vi "3458A Initiate Digitizing Process.vi"(8 "error in":errorcluster, 11 "session in":T1 {"channels"."Range [Vpk]" min=0.0}) -> (0 "error out":errorcluster, 3 "session out":T1 {"channels"."Range [Vpk]" min=0.0})   [LabVIEW 2018, in "3458A Virtual Digitizer.lvlib"]
doc: "Initiates acquisition for both single shot and streaming modes. It creates data queues and starts digitizing processes, one for each channel. If succeds the process immediatelly starts digitizing (after trigger event occures) and starts filling the queues with data. So this VI must be immediatelly followed by fetch loop that takes out data from the queue! This may be called repeatedely without calling 'Setup' function if multiple records are required with identical configuration."
uses:
  3458A Virtual Digitizer.lvlib
  3458A Digitizer Session.ctl
  3458A Virtual Channel Config.ctl
  Counter/Counter Session.ctl
  Counter/Counter Type.ctl
  AWG/AWG Session.ctl
  AWG/AWG Type.ctl
  3458A Sync Mode.ctl
  3458A Idn Mode.ctl
  3458A Digitizing Low Levels/Configure/Sampling Mode.ctl
  3458A Digitizing Process Options.ctl
  3458A Data Packet.ctl
  3458A Aux Record Data.ctl
  3458A Digitizing Low Levels/Configure/Level Setup.ctl
  3458A Digitizing Low Levels/Configure/First Sample Trigger.ctl
  3458A Aperture Selection Mode.ctl
  AWG/AWG.lvlib
  Counter/Counter.lvlib
  3458A Digitizing Low Levels/3458A Digitizing Low Levels.lvlib
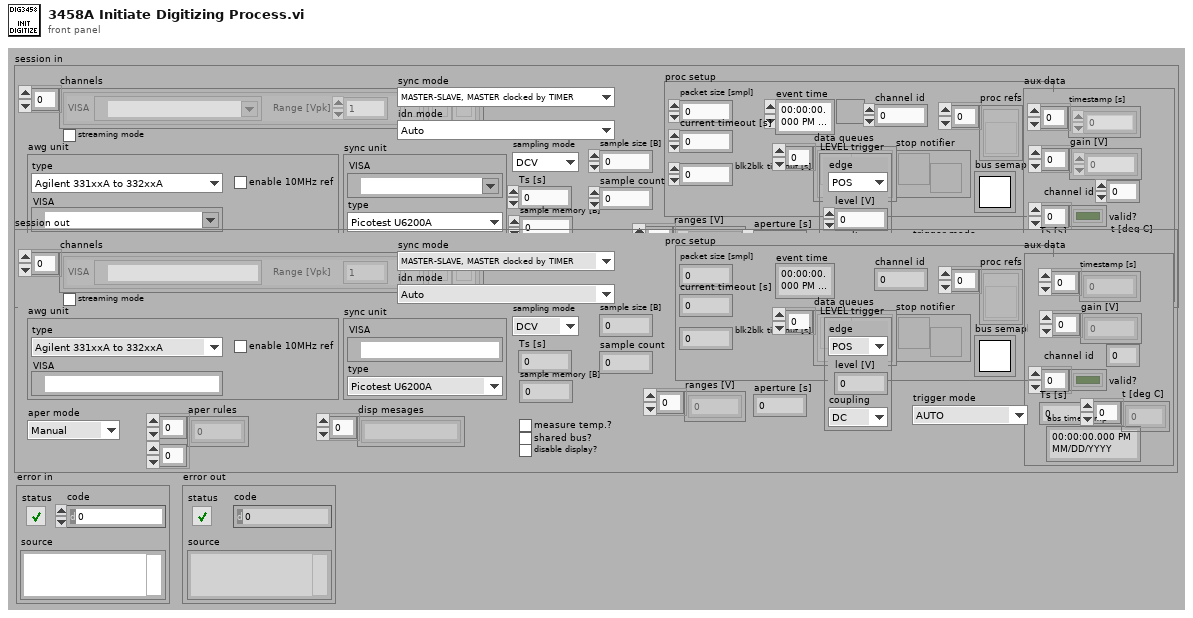
[diagram p1: front panel]
types:
  T1 = typedef "3458A Virtual Digitizer.lvlib/3458A Digitizer Session.ctl" = cluster{"channels":T2[], "sync unit":T3, "awg unit":T5, "sync mode":T7, "streaming mode":bool, "idn mode":T8, "sampling mode":T9, "Ts [s]":dbl, "sample memory [B]":i32, "proc setup":T10, "sample size [B]":i32, "sample count":i32, "aux data":T12, "ranges [V]":dbl[], "aperture [s]":dbl, "LEVEL trigger":T13, "trigger mode":T14, "measure temp.?":bool, "disp mesages":string[], "shared bus?":bool, "disable display?":bool, "aper mode":T15, "aper rules":dbl[][]}
  T2 = typedef "3458A Virtual Digitizer.lvlib/3458A Virtual Channel Config.ctl" = cluster{"VISA":refnum<visa-resource-name>, "Range [Vpk]":dbl, "btn clr":bool, "btn up":bool, "btn down":bool}
  T3 = typedef "Counter.lvlib/Counter Session.ctl" = cluster{"VISA":refnum<visa-resource-name>, "type":T4}
  T4 = typedef "Counter.lvlib/Counter Type.ctl" = enum16{"Picotest U6200A", "dummy"}
  T5 = typedef "AWG.lvlib/AWG Session.ctl" = cluster{"type":T6, "VISA":refnum<visa-resource-name>, "enable 10MHz ref":bool}
  T6 = typedef "AWG.lvlib/AWG Type.ctl" = enum16{"Agilent 331xxA to 332xxA", "Agilent 335xxA to 336xxA", "Tektronix AFG3101C", "dummy"}
  T7 = typedef "3458A Virtual Digitizer.lvlib/3458A Sync Mode.ctl" = enum16{"MASTER-SLAVE, MASTER clocked by TIMER", "MASTER-SLAVE, MASTER clocked by AWG", "ALL clocked by AWG", "MASTER-SLAVE, ALL clocked by TIMER", "ALL clocked by AWG with DFLL"}
  T8 = typedef "3458A Virtual Digitizer.lvlib/3458A Idn Mode.ctl" = enum16{"Auto", "Sequential (chn A, chn B, ...)", "From calibration string"}
  T9 = typedef "3458A Virtual Digitizer.lvlib/3458A Digitizing Low Levels.lvlib/Sampling Mode.ctl" = enum16{"DCV", "DSDC", "DSAC"}
  T10 = typedef "3458A Virtual Digitizer.lvlib/3458A Digitizing Process Options.ctl" = cluster{"channel id":i32, "packet size [smpl]":i32, "current timeout [s]":dbl, "blk2blk timeout [s]":dbl, "event time":timestamp, "stop notifier":refnum<notifier>, "data queues":refnum<queue>[], "proc refs":refnum<vi>[], "bus semaphore":T11}
  T11 = typedef "Semaphore RefNum" = refnum<k1>
  T12 = typedef "3458A Virtual Digitizer.lvlib/3458A Aux Record Data.ctl" = cluster{"channel id":i32, "valid?":bool[], "gain [V]":dbl[], "timestamp [s]":dbl[], "Ts [s]":dbl, "abs timestamp":timestamp, "t [deg C]":dbl[]}
  T13 = typedef "3458A Virtual Digitizer.lvlib/3458A Digitizing Low Levels.lvlib/Level Setup.ctl" = cluster{"edge":enum16{"POS", "NEG"}, "level [V]":dbl, "coupling":enum16{"DC", "AC"}}
  T14 = typedef "3458A Virtual Digitizer.lvlib/3458A Digitizing Low Levels.lvlib/First Sample Trigger.ctl" = enum16{"AUTO", "EXT", "SYN", "SGL", "HOLD", "LEVEL"}
  T15 = typedef "3458A Virtual Digitizer.lvlib/3458A Aperture Selection Mode.ctl" = enum16{"Manual", "Maximum", "Table"}
  T16 = typedef "3458A Virtual Digitizer.lvlib/3458A Data Packet.ctl" = cluster{"data":i32[][], "offset [smpl]":i32, "count [smpl]":i32, "all done?":bool, "sampling?":bool, "queue buffer [%]":dbl, "valid?":bool}
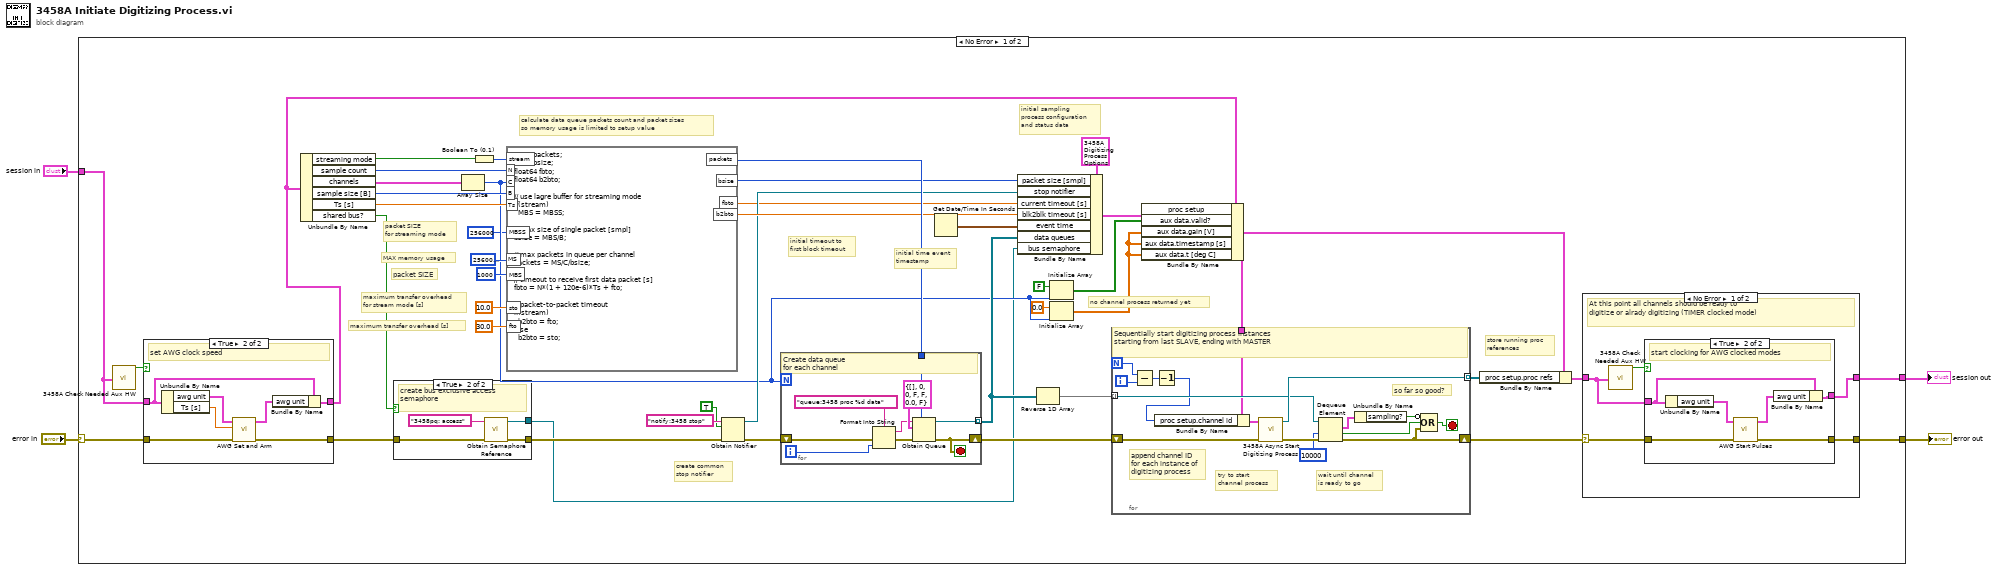
[diagram p0: block diagram]
diagram:
  n1 = case shown="No Error" "error in" {
    selector: "error in" -> [w8 w104]
    tunnel: [w24 w104] -> w4
    tunnel: "session in" -> [w7 w103]
    tunnel: [w23 w103] -> w2
    frame No Error {
      # "packet SIZE\nfor streaming mode"
      # "no channel process returned yet"
      # "initial time event\ntimestamp"
      # "maximum transfer overhead\nfor stream mode [s]"
      # "store running proc\nreferences"
      # "create common\nstop notifier"
      # "initial timeout to\nfirst block timeout"
      # "maximum transfer overhead [s]"
      # "initial sampling\nprocess configuration\nand status data"
      # "calculate data queue packets count and packet sizes\nso memory usage is limited to setup value"
      # "packet SIZE"
      # "MAX memory usage"
      n2 = call "3458A Check Needed Aux HW.vi"("digitizer session"=w7) -> ("uses AWG clocking?"=w6:bool)  [unwired: 13 in, 5 out]
      n3 = case shown="True" w6 {
        tunnel: w8 -> [w49 w57]
        tunnel: w7 -> [w50 w54]
        tunnel: [w49 w53] -> w9
        tunnel: [w50 w52] -> w5
        frame False {
          # "do nothing for TIMER clocked modes"
        }
        frame True {
          # "set AWG clock speed"
          n4 = Unbundle By Name(w54) -> ("awg unit"=w56:T5, "Ts [s]"=w51:dbl)
          n5 = call "AWG Set and Arm.vi"("error in (no error)"=w57, "T [s] (1ms)"=w51, "awg session in"=w56) -> ("error out"=w53:errorcluster, "awg session out"=w55:T5)  [unwired: 7 in]
          n6 = Bundle By Name(cluster=w54, "awg unit"=w55) -> (w52:T1)
        }
      }
      n7 = Unbundle By Name(w5) -> ("streaming mode"=w47:bool, "sample count"=w45:i32, "channels"=w44:T2[], "sample size [B]"=w22:i32, "Ts [s]"=w21:dbl, "shared bus?"=w12:bool)
      n8 = case shown="True" w12 {
        tunnel: w9 -> [w58 w62]
        tunnel: [w58 w61] -> w13
        tunnel: [_ w59] -> w11
        frame False {
        }
        frame True {
          # "create bus exclusive access\nsemaphore"
          n9 = call <vilib>:"Obtain Semaphore Reference.vi"("error in (no error)"=w62, "name (unnamed)"="3458pq: access") -> ("error out"=w61:errorcluster, "semaphore"=w59:T11)  [unwired: 3 in, 1 out]
        }
      }
      n10 = Array Size(array=w44) -> (size(s)=w15:i32)
      n11 = Boolean To (0,1)(Boolean=w47) -> (0, 1=w46:i16)
      n12 = formula code="int32 packets;\nint32 bsize;\nfloat64 fbto;\nfloat64 b2bto;\n\n// use lagre buffer for streaming mode\nif(stream)\n  MBS = MBSS;\n\n// max size of single packet [smpl]\nbsize = MBS/B;\n\n// max packets in queue per channel\npackets = MS/C/bsize;\n\n// timeout to receive first data packet [s]\nfbto = N*(1 + 120e-6)*Ts + fto;\n\n// packet-to-packet timeout\nif(stream)\n  b2bto = fto;\nelse\n  b2bto = sto;"("stream"=w46, "N"=w45, "C"=w15, "MS"=256000000 ("y"), "MBS"=1000 ("y"), "Ts"=w21, "fto"=30.0 ("input variable"), "B"=w22, "sto"=10.0 ("input variable"), "MBSS"=256000 ("y")) -> ("packets"=w41:i32, "bsize"=w40:i32, "fbto"=w19:dbl, "b2bto"=w36:dbl)
      n13 = Obtain Notifier(name (unnamed)="notify:3458 stop", notification data type=TRUE, error in (no error)=w13) -> (notifier out=w32:refnum<notifier>, error out=w34:errorcluster)  [unwired: 1 in, 1 out]
      n14 = for {
        N: w15 -> [_]
        tunnel: w41 -> [w102]
        shift-right: [w94] -> w39
        shift-left: w34 -> [w99]
        tunnel: [w100] -> w29 mode=indexing
        i -> [w95]
        stop <- w94 stop-if-true
        # "Create data queue\nfor each channel"
        n15 = Format Into String(format string="queue:3458 proc %d data" ("name (unnamed)"), error in=w99, w95) -> (resulting string=w97:string, error out=w98:errorcluster)  [unwired: 1 in]
        n16 = Obtain Queue(max queue size (-1, unlimited)=w102, name (unnamed)=w97, element data type=T16 {"data"=[], "offset [smpl]"=0, "count [smpl]"=0, "all done?"=FALSE, "sampling?"=FALSE, "queue buffer [%]"=0.0, "valid?"=FALSE} ("niScope packet"), error in (no error)=w98) -> (queue out=w100:refnum<queue>, error out=w94:errorcluster)  [unwired: 1 in, 1 out]
      }
      n17 = Get Date/Time In Seconds() -> (seconds since 1Jan1904=w37:timestamp)
      n18 = Bundle By Name(cluster=T10 {"channel id"=0, "packet size [smpl]"=0, "current timeout [s]"=0.0, "blk2blk timeout [s]"=0.0, "event time"=timestamp(0 s since 1904-01-01), "stop notifier"=refnum, "data queues"=[], "proc refs"=[], "bus semaphore"=refnum} ("setup"), "packet size [smpl]"=w40, "stop notifier"=w32, "current timeout [s]"=w19, "blk2blk timeout [s]"=w36, "event time"=w37, "data queues"=w29, "bus semaphore"=w11) -> (w31:T10)
      n19 = Reverse 1D Array(array=w29) -> (reversed array=w30:refnum<queue>[])
      n20 = Initialize Array(FALSE, w15) -> (w18:bool[])
      n21 = Initialize Array(0.0, w15) -> (w14:dbl[])
      n22 = Bundle By Name(cluster=w5, "proc setup"=w31, "aux data.valid?"=w18, "aux data.gain [V]"=w14, "aux data.timestamp [s]"=w14, "aux data.t [deg C]"=w14) -> (w27:T1)
      n23 = for {
        N -> [w86]
        tunnel: [w92] -> w26 mode=indexing
        tunnel: w27 -> [w87]
        tunnel: w30 -> [w90] mode=indexing
        shift-right: [w82] -> w28
        shift-left: w39 -> [w93]
        i -> [w85]
        stop <- w80 stop-if-true
        # "so far so good?"
        # "wait until channel\nis ready to go"
        # "try to start\nchannel process"
        # "append channel ID\nfor each instance of\ndigitizing process"
        # "Sequentially start digitizing process instances\nstarting from last SLAVE, ending with MASTER"
        n24 = Subtract(x=w86, y=w85) -> (x-y=w84:i32)
        n25 = Decrement(x=w84) -> (x-1=w83:i32)
        n26 = Bundle By Name(cluster=w87, "proc setup.channel id"=w83) -> (w88:T1)
        n27 = call "3458A Async Start Digitizing Process.vi"("error in"=w93, "digitizer session"=w88) -> ("error out"=w91:errorcluster, "vi ref out"=w92:refnum<vi>)  [unwired: 8 in]
        n28 = Dequeue Element(queue=w90, timeout in ms (-1)=10000, error in (no error)=w91) -> (element=w79:T16, timed out?=w81:bool, error out=w82:errorcluster)  [unwired: 1 out]
        n29 = Unbundle By Name(w79) -> ("sampling?"=w78:bool)
        n30 = Compound Arithmetic op=OR(invert w78, w81, w82) -> (w80:bool)
      }
      n31 = Bundle By Name(cluster=w27, "proc setup.proc refs"=w26) -> (w25:T1)
      n32 = case shown="No Error" w28 {
        selector: w28 -> [w66 w77]
        tunnel: w25 -> [w65 w76]
        tunnel: [w64 w77] -> w24
        tunnel: [w63 w76] -> w23
        frame No Error {
          # "At this point all channels should be ready to\ndigitize or alrady digitizing (TIMER clocked mode)"
          n33 = call "3458A Check Needed Aux HW.vi"("digitizer session"=w65) -> ("uses AWG clocking?"=w67:bool)  [unwired: 13 in, 5 out]
          n34 = case shown="True" w67 {
            tunnel: w66 -> [w68 w75]
            tunnel: w65 -> [w69 w72]
            tunnel: [w68 w71] -> w64
            tunnel: [w69 w70] -> w63
            frame False {
              # "do nothing for TIMER clocked modes"
            }
            frame True {
              # "start clocking for AWG clocked modes"
              n35 = Unbundle By Name(w72) -> ("awg unit"=w74:T5)
              n36 = call "AWG Start Pulses.vi"("error in (no error)"=w75, "awg session in"=w74) -> ("error out"=w71:errorcluster, "awg session out"=w73:T5)  [unwired: 8 in]
              n37 = Bundle By Name(cluster=w72, "awg unit"=w73) -> (w70:T1)
            }
          }
        }
        frame Error {
        }
      }
    }
    frame Error {
    }
  }
  "error out" <- w4
  "session out" <- w2
